vi "UTL_ JL Scaling Calculation.vi"(8 "Error":errorcluster, 11 "Scaling Parameters":T2) -> (0 "Error Out":errorcluster, 3 "Scaling Factors Out":T1)   [LabVIEW 2023]
doc: "Calculates scaled value given raw value and scaling parameters."
uses:
  Controls/Cluster_JL Scaling Control.ctl
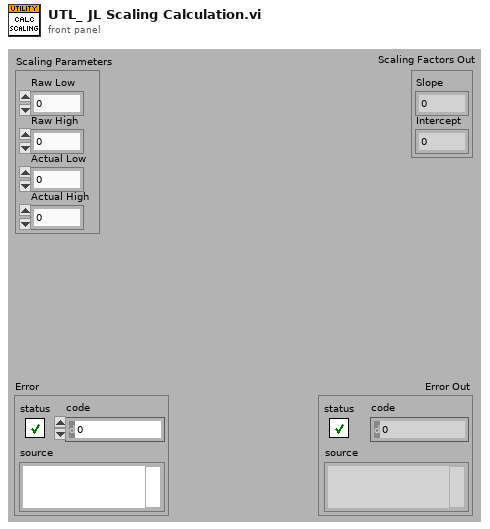
[diagram p1: front panel]
types:
  T1 = typedef "Cluster_JL Scaling Control.ctl" = cluster{"Slope":dbl, "Intercept":dbl}
  T2 = cluster{"Raw Low":dbl, "Raw High":dbl, "Actual Low":dbl, "Actual High":dbl}
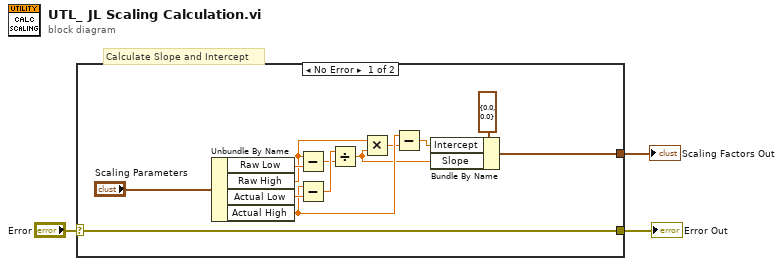
[diagram p0: block diagram]
diagram:
  # "Calculate Slope and Intercept"
  n1 = case shown="No Error" "Error" {
    selector: "Error" -> [w16 w17]
    tunnel: [w16 w17] -> w2
    tunnel: [w4 _] -> w1
    frame No Error {
      n2 = Unbundle By Name("Scaling Parameters") -> ("Raw Low"=w14:dbl, "Raw High"=w13:dbl, "Actual Low"=w12:dbl, "Actual High"=w11:dbl)
      n3 = Subtract(x=w13, y=w14) -> (x-y=w9:dbl)
      n4 = Subtract(x=w11, y=w12) -> (x-y=w10:dbl)
      n5 = Divide(x=w10, y=w9) -> (x/y=w7:dbl)
      n6 = Multiply(x=w13, y=w7) -> (x*y=w6:dbl)
      n7 = Subtract(x=w11, y=w6) -> (x-y=w5:dbl)
      n8 = Bundle By Name(cluster=T1 {"Slope"=0.0, "Intercept"=0.0} ("Scaling Factors Out"), "Intercept"=w5, "Slope"=w7) -> (w4:T1)
    }
    frame Error {
    }
  }
  "Error Out" <- w2
  "Scaling Factors Out" <- w1
